vi "Autonomous Independent.vi"() -> ()   [LabVIEW 2013]
doc: "This VI is called when autonomous begins, and will automatically be terminated when autonomous ends. You can carry out timed or sensor driven robot movement independently without needing to return to the caller."
uses:
  Robot Global Data.vi
  <vilib>/Rock Robotics/WPI/RobotDrive/WPI_RobotDriveArcadeDrive_Standard(NoSaturation).vi
panel:
  out "Limit Switch":bool
  out "Light on if Arm is Down/Going Down":bool
  out "Intake pneumatics":bool
  out "Drive Right Motor":dbl
  out "Drive Left Motor":dbl
  # "Be sure to right-click and choose Data Operations>>Make Current Value default if you want to save the array values with the VI"
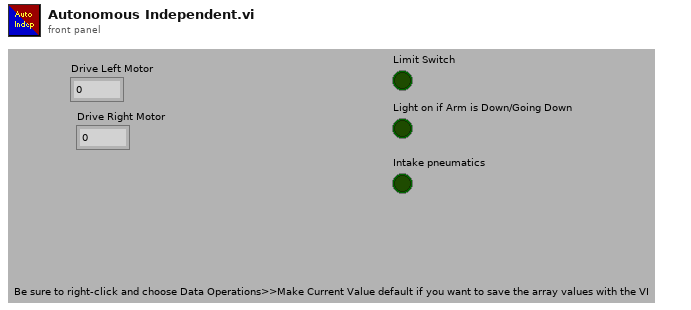
[diagram p1: front panel]
types:
  T1 = typedef "WPI_RobotDriveDevRef.ctl" = cluster{"DevStatus":errorcluster, "Motors[]":T2[], "Square Inputs":bool, "Max Output":dbl, "Isochronous":bool}
  T2 = typedef "WPI_MotorControlDeviceRef.ctl" = cluster{"DeviceStatus":errorcluster, "Type":enum16{"PWM", "CAN"}, "PWM":cluster{"Digital Module":T3, "PWM Channel":T4, "DeadBand":T5}, "CAN":cluster{"Device Number":u8, "Control Mode":T6, "Semaphore":T7, "Max Vout":dbl}, "Invert":bool, "TransformRef":T8, "InvTransformRef":T8}
  T3 = typedef "FPGA_TypedefDigitalModule.ctl" = enum16{"Digital Module 1", "Digital Module 2"}
  T4 = typedef "FPGA_DIOPWMChannel.ctl" = enum8{"PWM 1", "PWM 2", "PWM 3", "PWM 4", "PWM 5", "PWM 6", "PWM 7", "PWM 8", "PWM 9", "PWM 10", "Invalid"}
  T5 = typedef "WPI_PWMDeadband.ctl" = cluster{"Name":string, "maxPositivePwm":i32, "minPositivePwm":i32, "centerPwm":i32, "maxNegativePwm":i32, "minNegativePwm":i32, "angularRange":u16}
  T6 = typedef "WPI_CANJaguar_ControlMode.ctl" = enum8{"Percent VBus", "Current", "Speed", "Position", "Voltage"}
  T7 = typedef "Semaphore RefNum" = refnum<k1>
  T8 = typedef "WPI_PWMTransform_ConPane.ctl" = refnum<vi>
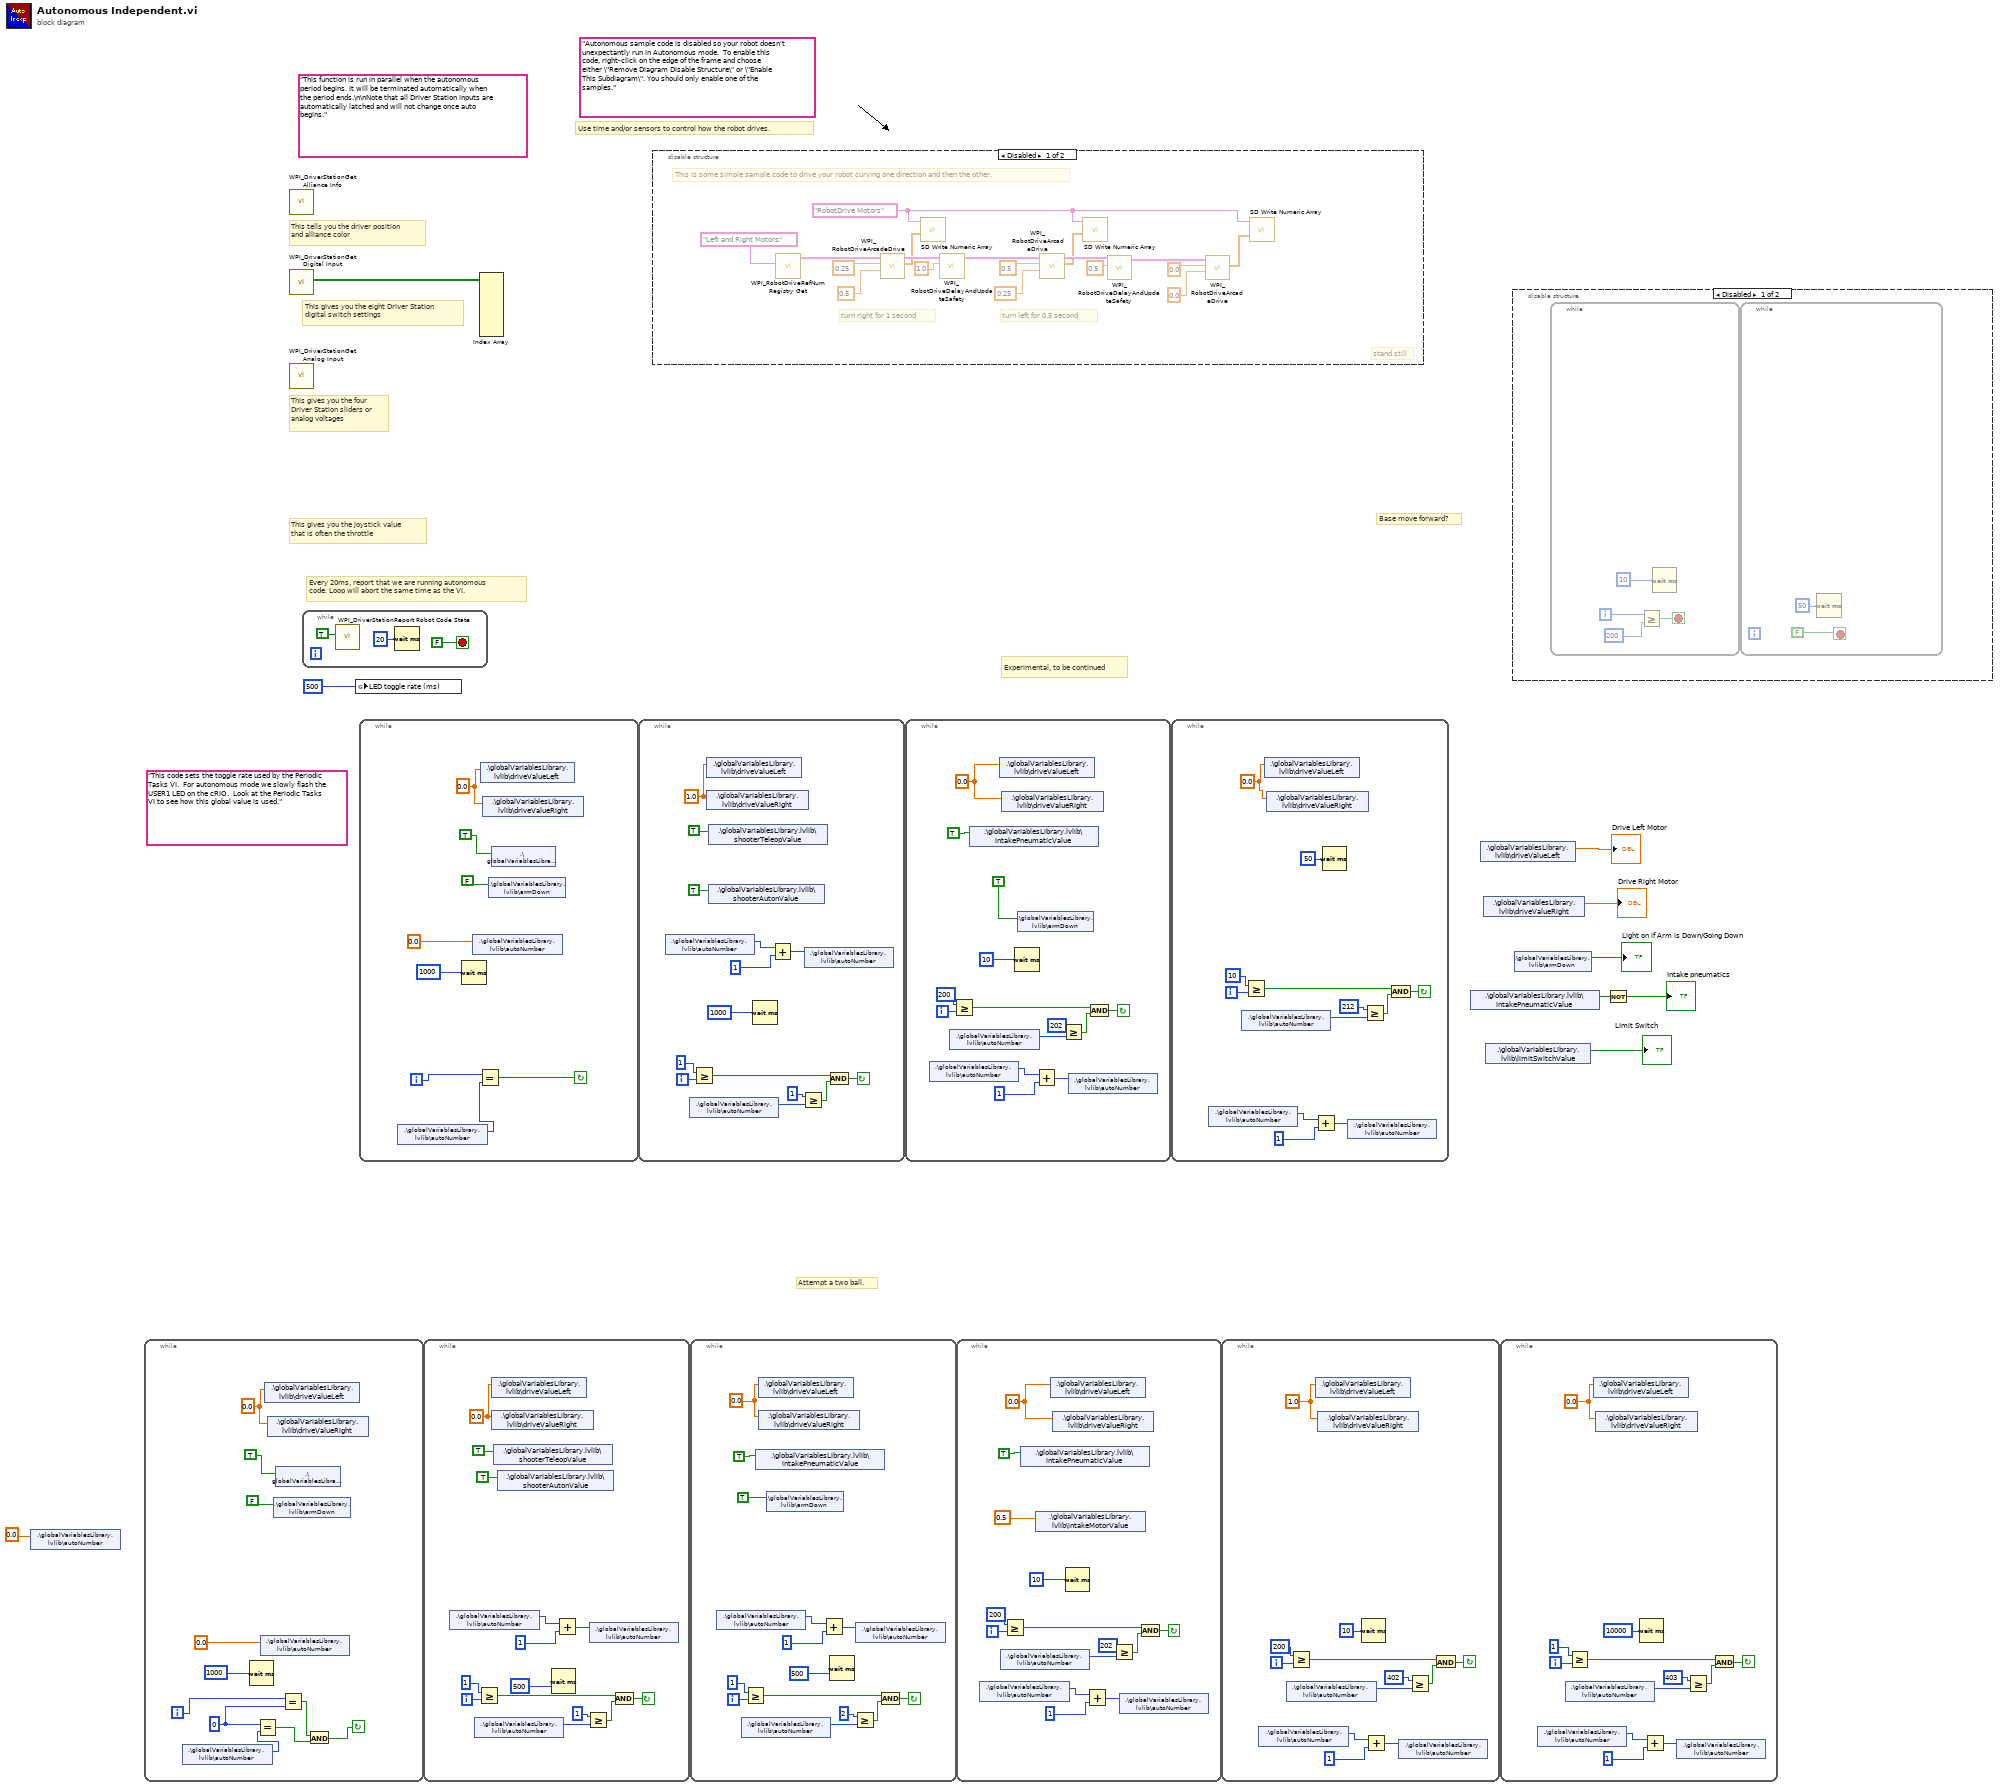
[diagram p0: block diagram]
diagram:
  (unwired) "This code sets the toggle rate used by the Periodic Tasks VI.  For autonomous mode we slowly flash the USER1 LED on the cRIO.  Look at the Periodic Tasks VI to see how this global value is used."
  (unwired) "Autonomous sample code is disabled so your robot doesn't unexpectantly run in Autonomous mode.  To enable this code, right-click on the edge of the frame and choose either \"Remove Diagram Disable Structure\" or \"Enable This Subdiagram\". You should only enable one of the samples."
  (unwired) "This function is run in parallel when the autonomous period begins. It will be terminated automatically when the period ends.\n\nNote that all Driver Station inputs are automatically latched and will not change once auto begins."
  # "Attempt a two ball."
  # "Base move forward?"
  # "Experimental, to be continued"
  # "Every 20ms, report that we are running autonomous\ncode. Loop will abort the same time as the VI."
  # "This gives you the joystick value\nthat is often the throttle"
  # "Use time and/or sensors to control how the robot drives."
  # "This tells you the driver position\nand alliance color"
  # "This gives you the eight Driver Station\ndigital switch settings"
  # "This gives you the four\nDriver Station sliders or\nanalog voltages"
  n1 = shared-variable ".\\globalVariablesLibrary.lvlib\\autoNumber"(0.0) -> ()  [unwired: 1 in, 1 out]
  n2 = while {
    i -> [w13]
    stop <- w14 continue-if-true
    w11 = 0
    w19 = 0.0
    n3 = shared-variable ".\\globalVariablesLibrary.lvlib\\autoNumber"() -> (w15:i16)  [unwired: 1 in, 1 out]
    n4 = Wait (ms)(milliseconds to wait=u32 1000) -> ()  [unwired: 1 out]
    n5 = Equal?(x=w11, y=w15) -> (x = y?=w10:bool)
    n6 = shared-variable ".\\globalVariablesLibrary.lvlib\\autoNumber"(0.0) -> ()  [unwired: 1 in, 1 out]
    n7 = shared-variable ".\\globalVariablesLibrary.lvlib\\driveValueLeft"(w19) -> ()  [unwired: 1 in, 1 out]
    n8 = shared-variable ".\\globalVariablesLibrary.lvlib\\driveValueRight"(w19) -> ()  [unwired: 1 in, 1 out]
    n9 = shared-variable ".\\globalVariablesLibrary.lvlib\\armDown"(FALSE) -> ()  [unwired: 1 in, 1 out]
    n10 = shared-variable ".\\globalVariablesLibrary.lvlib\\armUp"(TRUE) -> ()  [unwired: 1 in, 1 out]
    n11 = Equal?(x=w13, y=w11) -> (x = y?=w12:bool)
    n12 = And(x=w12, y=w10) -> (x .and. y?=w14:bool)
  }
  n13 = call <vilib>:"WPI_DriverStationGet Alliance Info.vi"() -> ()  [unwired: 12 out]
  n14 = call <vilib>:"WPI_DriverStationGet Digital Input.vi"() -> ("Driver Station Digital Input (1-8)"=w9:bool[])  [unwired: 11 out]
  n15 = call <vilib>:"WPI_DriverStationGet Analog Input.vi"() -> ()  [unwired: 12 out]
  n16 = while {
    stop <- FALSE stop-if-true
    n17 = call <vilib>:"WPI_DriverStationReport Robot Code State.vi"("Autonomous"=TRUE) -> ()  [unwired: 10 in, 1 out]
    n18 = Wait (ms)(milliseconds to wait=u32 20) -> ()  [unwired: 1 out]
  }
  n19 = global write "Robot Global Data.vi" "LED toggle rate (ms)"(u32 500 ("LED ms toggle rate")) -> ()
  n20 = while {
    i -> [w25]
    stop <- w24 continue-if-true
    w30 = 0.0
    n21 = shared-variable ".\\globalVariablesLibrary.lvlib\\autoNumber"() -> (w26:i16)  [unwired: 1 in, 1 out]
    n22 = Wait (ms)(milliseconds to wait=u32 1000) -> ()  [unwired: 1 out]
    n23 = shared-variable ".\\globalVariablesLibrary.lvlib\\autoNumber"(0.0) -> ()  [unwired: 1 in, 1 out]
    n24 = Equal?(x=w25, y=w26) -> (x = y?=w24:bool)
    n25 = shared-variable ".\\globalVariablesLibrary.lvlib\\driveValueLeft"(w30) -> ()  [unwired: 1 in, 1 out]
    n26 = shared-variable ".\\globalVariablesLibrary.lvlib\\driveValueRight"(w30) -> ()  [unwired: 1 in, 1 out]
    n27 = shared-variable ".\\globalVariablesLibrary.lvlib\\armDown"(FALSE) -> ()  [unwired: 1 in, 1 out]
    n28 = shared-variable ".\\globalVariablesLibrary.lvlib\\armUp"(TRUE) -> ()  [unwired: 1 in, 1 out]
  }
  n29 = while {
    i -> [w35]
    stop <- w32 continue-if-true
    w42 = 0.0
    n30 = shared-variable ".\\globalVariablesLibrary.lvlib\\autoNumber"() -> (w41:i16)  [unwired: 1 in, 1 out]
    n31 = shared-variable ".\\globalVariablesLibrary.lvlib\\autoNumber"() -> (w38:i16)  [unwired: 1 in, 1 out]
    n32 = Greater Or Equal?(x=1, y=w35) -> (x >= y?=w33:bool)
    n33 = shared-variable ".\\globalVariablesLibrary.lvlib\\driveValueLeft"(w42) -> ()  [unwired: 1 in, 1 out]
    n34 = shared-variable ".\\globalVariablesLibrary.lvlib\\driveValueRight"(w42) -> ()  [unwired: 1 in, 1 out]
    n35 = shared-variable ".\\globalVariablesLibrary.lvlib\\shooterTeleopValue"(TRUE) -> ()  [unwired: 1 in, 1 out]
    n36 = shared-variable ".\\globalVariablesLibrary.lvlib\\shooterAutonValue"(TRUE) -> ()  [unwired: 1 in, 1 out]
    n37 = Wait (ms)(milliseconds to wait=u32 500) -> ()  [unwired: 1 out]
    n38 = Add(x=w41, y=1) -> (x+y=w40:i32)
    n39 = Greater Or Equal?(x=1, y=w38) -> (x >= y?=w36:bool)
    n40 = shared-variable ".\\globalVariablesLibrary.lvlib\\autoNumber"(w40) -> ()  [unwired: 1 in, 1 out]
    n41 = And(x=w33, y=w36) -> (x .and. y?=w32:bool)
  }
  n42 = Index Array(array=w9) -> ()  [unwired: 8 in, 8 out]
  n43 = while {
    i -> [w49]
    stop <- w46 continue-if-true
    w56 = 1.0
    n44 = shared-variable ".\\globalVariablesLibrary.lvlib\\autoNumber"() -> (w55:i16)  [unwired: 1 in, 1 out]
    n45 = shared-variable ".\\globalVariablesLibrary.lvlib\\autoNumber"() -> (w52:i16)  [unwired: 1 in, 1 out]
    n46 = Greater Or Equal?(x=1, y=w49) -> (x >= y?=w47:bool)
    n47 = shared-variable ".\\globalVariablesLibrary.lvlib\\driveValueLeft"(w56) -> ()  [unwired: 1 in, 1 out]
    n48 = shared-variable ".\\globalVariablesLibrary.lvlib\\driveValueRight"(w56) -> ()  [unwired: 1 in, 1 out]
    n49 = shared-variable ".\\globalVariablesLibrary.lvlib\\shooterTeleopValue"(TRUE) -> ()  [unwired: 1 in, 1 out]
    n50 = shared-variable ".\\globalVariablesLibrary.lvlib\\shooterAutonValue"(TRUE) -> ()  [unwired: 1 in, 1 out]
    n51 = Wait (ms)(milliseconds to wait=u32 1000) -> ()  [unwired: 1 out]
    n52 = Add(x=w55, y=1) -> (x+y=w54:i32)
    n53 = Greater Or Equal?(x=1, y=w52) -> (x >= y?=w50:bool)
    n54 = shared-variable ".\\globalVariablesLibrary.lvlib\\autoNumber"(w54) -> ()  [unwired: 1 in, 1 out]
    n55 = And(x=w47, y=w50) -> (x .and. y?=w46:bool)
  }
  n56 = disable-structure shown="Disabled" {
    frame Disabled {
      w60 = "RobotDrive Motors" ("Name")
      # "This is some simple sample code to drive your robot curving one direction and then the other."
      # "stand still"
      # "turn left for 0.5 second"
      # "turn right for 1 second"
      n57 = call <vilib>:"WPI_RobotDriveRefNum Registry Get.vi"("refnum name"="Left and Right Motors") -> ("RobotDriveDevRef"=w64:T1)  [unwired: 1 in, 9 out]
      n58 = call-poly <vilib>:"WPI_RobotDriveArcadeDrive.vi"("Y axis value"=0.5 ("X axis value"), "X axis value"=0.25, "RobotDriveDevRef"=w64) -> ("Motor Values"=w63:dbl[], "RobotDriveDevRef"=w71:T1)  [unwired: 1 in, 6 out]
      n59 = call <vilib>:"SD Write Numeric Array.vi"("Numeric Array"=w63, "Name"=w60) -> ()  [unwired: 8 in, 2 out]
      n60 = call <vilib>:"WPI_RobotDriveDelayAndUpdateSafety.vi"("Delay (s)"=1.0, "RobotDriveDevRef"=w71) -> ("RobotDriveDevRef 2"=w70:T1)  [unwired: 8 in, 1 out]
      n61 = call-poly <vilib>:"WPI_RobotDriveArcadeDrive.vi"("Y axis value"=0.25 ("X axis value"), "X axis value"=0.5, "RobotDriveDevRef"=w70) -> ("Motor Values"=w62:dbl[], "RobotDriveDevRef"=w69:T1)  [unwired: 1 in, 6 out]
      n62 = call <vilib>:"SD Write Numeric Array.vi"("Numeric Array"=w62, "Name"=w60) -> ()  [unwired: 8 in, 2 out]
      n63 = call <vilib>:"WPI_RobotDriveDelayAndUpdateSafety.vi"("Delay (s)"=0.5, "RobotDriveDevRef"=w69) -> ("RobotDriveDevRef 2"=w68:T1)  [unwired: 8 in, 1 out]
      n64 = call-poly <vilib>:"WPI_RobotDriveArcadeDrive.vi"("Y axis value"=0.0 ("X axis value"), "X axis value"=0.0, "RobotDriveDevRef"=w68) -> ("Motor Values"=w61:dbl[])  [unwired: 1 in, 7 out]
      n65 = call <vilib>:"SD Write Numeric Array.vi"("Numeric Array"=w61, "Name"=w60) -> ()  [unwired: 8 in, 2 out]
    }
    frame Enabled {
    }
  }
  n66 = while {
    i -> [w83]
    stop <- w80 continue-if-true
    w90 = 0.0
    n67 = shared-variable ".\\globalVariablesLibrary.lvlib\\autoNumber"() -> (w89:i16)  [unwired: 1 in, 1 out]
    n68 = shared-variable ".\\globalVariablesLibrary.lvlib\\autoNumber"() -> (w86:i16)  [unwired: 1 in, 1 out]
    n69 = Greater Or Equal?(x=1, y=w83) -> (x >= y?=w81:bool)
    n70 = shared-variable ".\\globalVariablesLibrary.lvlib\\intakePneumaticValue"(TRUE) -> ()  [unwired: 1 in, 1 out]
    n71 = shared-variable ".\\globalVariablesLibrary.lvlib\\driveValueLeft"(w90) -> ()  [unwired: 1 in, 1 out]
    n72 = shared-variable ".\\globalVariablesLibrary.lvlib\\driveValueRight"(w90) -> ()  [unwired: 1 in, 1 out]
    n73 = shared-variable ".\\globalVariablesLibrary.lvlib\\armDown"(TRUE) -> ()  [unwired: 1 in, 1 out]
    n74 = Add(x=w89, y=1) -> (x+y=w88:i32)
    n75 = Wait (ms)(milliseconds to wait=u32 500) -> ()  [unwired: 1 out]
    n76 = Greater Or Equal?(x=2, y=w86) -> (x >= y?=w84:bool)
    n77 = shared-variable ".\\globalVariablesLibrary.lvlib\\autoNumber"(w88) -> ()  [unwired: 1 in, 1 out]
    n78 = And(x=w81, y=w84) -> (x .and. y?=w80:bool)
  }
  n79 = while {
    i -> [w96]
    stop <- w95 continue-if-true
    w103 = 0.0 ("Output")
    n80 = shared-variable ".\\globalVariablesLibrary.lvlib\\autoNumber"() -> (w94:i16)  [unwired: 1 in, 1 out]
    n81 = shared-variable ".\\globalVariablesLibrary.lvlib\\autoNumber"() -> (w101:i16)  [unwired: 1 in, 1 out]
    n82 = Greater Or Equal?(x=200, y=w96) -> (x >= y?=w97:bool)
    n83 = shared-variable ".\\globalVariablesLibrary.lvlib\\intakePneumaticValue"(TRUE) -> ()  [unwired: 1 in, 1 out]
    n84 = shared-variable ".\\globalVariablesLibrary.lvlib\\driveValueLeft"(w103) -> ()  [unwired: 1 in, 1 out]
    n85 = shared-variable ".\\globalVariablesLibrary.lvlib\\driveValueRight"(w103) -> ()  [unwired: 1 in, 1 out]
    n86 = Wait (ms)(milliseconds to wait=u32 10) -> ()  [unwired: 1 out]
    n87 = shared-variable ".\\globalVariablesLibrary.lvlib\\armDown"(TRUE) -> ()  [unwired: 1 in, 1 out]
    n88 = Add(x=w94, y=1) -> (x+y=w93:i32)
    n89 = Greater Or Equal?(x=202, y=w101) -> (x >= y?=w99:bool)
    n90 = shared-variable ".\\globalVariablesLibrary.lvlib\\autoNumber"(w93) -> ()  [unwired: 1 in, 1 out]
    n91 = And(x=w97, y=w99) -> (x .and. y?=w95:bool)
  }
  n92 = while {
    i -> [w111]
    stop <- w110 continue-if-true
    w117 = 0.0 ("Output")
    n93 = shared-variable ".\\globalVariablesLibrary.lvlib\\autoNumber"() -> (w109:i16)  [unwired: 1 in, 1 out]
    n94 = shared-variable ".\\globalVariablesLibrary.lvlib\\autoNumber"() -> (w116:i16)  [unwired: 1 in, 1 out]
    n95 = Greater Or Equal?(x=200, y=w111) -> (x >= y?=w112:bool)
    n96 = shared-variable ".\\globalVariablesLibrary.lvlib\\intakePneumaticValue"(TRUE) -> ()  [unwired: 1 in, 1 out]
    n97 = shared-variable ".\\globalVariablesLibrary.lvlib\\intakeMotorValue"(0.5) -> ()  [unwired: 1 in, 1 out]
    n98 = shared-variable ".\\globalVariablesLibrary.lvlib\\driveValueLeft"(w117) -> ()  [unwired: 1 in, 1 out]
    n99 = shared-variable ".\\globalVariablesLibrary.lvlib\\driveValueRight"(w117) -> ()  [unwired: 1 in, 1 out]
    n100 = Wait (ms)(milliseconds to wait=u32 10) -> ()  [unwired: 1 out]
    n101 = Add(x=w109, y=1) -> (x+y=w108:i32)
    n102 = Greater Or Equal?(x=202, y=w116) -> (x >= y?=w114:bool)
    n103 = shared-variable ".\\globalVariablesLibrary.lvlib\\autoNumber"(w108) -> ()  [unwired: 1 in, 1 out]
    n104 = And(x=w112, y=w114) -> (x .and. y?=w110:bool)
  }
  n105 = while {
    i -> [w123]
    stop <- w124 continue-if-true
    w130 = 0.0
    n106 = shared-variable ".\\globalVariablesLibrary.lvlib\\autoNumber"() -> (w122:i16)  [unwired: 1 in, 1 out]
    n107 = shared-variable ".\\globalVariablesLibrary.lvlib\\autoNumber"() -> (w129:i16)  [unwired: 1 in, 1 out]
    n108 = Greater Or Equal?(x=10, y=w123) -> (x >= y?=w125:bool)
    n109 = shared-variable ".\\globalVariablesLibrary.lvlib\\driveValueLeft"(w130) -> ()  [unwired: 1 in, 1 out]
    n110 = shared-variable ".\\globalVariablesLibrary.lvlib\\driveValueRight"(w130) -> ()  [unwired: 1 in, 1 out]
    n111 = Add(x=w122, y=1) -> (x+y=w121:i32)
    n112 = Wait (ms)(milliseconds to wait=u32 50) -> ()  [unwired: 1 out]
    n113 = shared-variable ".\\globalVariablesLibrary.lvlib\\autoNumber"(w121) -> ()  [unwired: 1 in, 1 out]
    n114 = Greater Or Equal?(x=212, y=w129) -> (x >= y?=w127:bool)
    n115 = And(x=w125, y=w127) -> (x .and. y?=w124:bool)
  }
  n116 = while {
    i -> [w135]
    stop <- w136 continue-if-true
    w142 = 1.0
    n117 = shared-variable ".\\globalVariablesLibrary.lvlib\\autoNumber"() -> (w134:i16)  [unwired: 1 in, 1 out]
    n118 = shared-variable ".\\globalVariablesLibrary.lvlib\\autoNumber"() -> (w141:i16)  [unwired: 1 in, 1 out]
    n119 = Greater Or Equal?(x=200, y=w135) -> (x >= y?=w137:bool)
    n120 = shared-variable ".\\globalVariablesLibrary.lvlib\\driveValueLeft"(w142) -> ()  [unwired: 1 in, 1 out]
    n121 = shared-variable ".\\globalVariablesLibrary.lvlib\\driveValueRight"(w142) -> ()  [unwired: 1 in, 1 out]
    n122 = Wait (ms)(milliseconds to wait=u32 10) -> ()  [unwired: 1 out]
    n123 = Add(x=w134, y=1) -> (x+y=w133:i32)
    n124 = shared-variable ".\\globalVariablesLibrary.lvlib\\autoNumber"(w133) -> ()  [unwired: 1 in, 1 out]
    n125 = Greater Or Equal?(x=402, y=w141) -> (x >= y?=w139:bool)
    n126 = And(x=w137, y=w139) -> (x .and. y?=w136:bool)
  }
  n127 = shared-variable ".\\globalVariablesLibrary.lvlib\\intakePneumaticValue"() -> (w4:bool)  [unwired: 1 in, 1 out]
  n128 = shared-variable ".\\globalVariablesLibrary.lvlib\\driveValueLeft"() -> (→"Drive Left Motor":dbl)  [unwired: 1 in, 1 out]
  n129 = shared-variable ".\\globalVariablesLibrary.lvlib\\driveValueRight"() -> (→"Drive Right Motor":dbl)  [unwired: 1 in, 1 out]
  n130 = shared-variable ".\\globalVariablesLibrary.lvlib\\limitSwitchValue"() -> (→"Limit Switch":bool)  [unwired: 1 in, 1 out]
  n131 = while {
    i -> [w147]
    stop <- w148 continue-if-true
    w154 = 0.0
    n132 = shared-variable ".\\globalVariablesLibrary.lvlib\\autoNumber"() -> (w146:i16)  [unwired: 1 in, 1 out]
    n133 = shared-variable ".\\globalVariablesLibrary.lvlib\\autoNumber"() -> (w153:i16)  [unwired: 1 in, 1 out]
    n134 = Greater Or Equal?(x=1, y=w147) -> (x >= y?=w149:bool)
    n135 = shared-variable ".\\globalVariablesLibrary.lvlib\\driveValueLeft"(w154) -> ()  [unwired: 1 in, 1 out]
    n136 = shared-variable ".\\globalVariablesLibrary.lvlib\\driveValueRight"(w154) -> ()  [unwired: 1 in, 1 out]
    n137 = Wait (ms)(milliseconds to wait=u32 10000) -> ()  [unwired: 1 out]
    n138 = Add(x=w146, y=1) -> (x+y=w145:i32)
    n139 = shared-variable ".\\globalVariablesLibrary.lvlib\\autoNumber"(w145) -> ()  [unwired: 1 in, 1 out]
    n140 = Greater Or Equal?(x=403, y=w153) -> (x >= y?=w151:bool)
    n141 = And(x=w149, y=w151) -> (x .and. y?=w148:bool)
  }
  n142 = disable-structure shown="Disabled" {
    frame Disabled {
      n143 = while {
        i -> [w160]
        stop <- w158 stop-if-true
        n144 = Greater Or Equal?(x=w160, y=200) -> (x >= y?=w158:bool)
        n145 = Wait (ms)(milliseconds to wait=u32 10) -> ()  [unwired: 1 out]
      }
      n146 = while {
        stop <- FALSE stop-if-true
        n147 = Wait (ms)(milliseconds to wait=u32 50) -> ()  [unwired: 1 out]
      }
    }
    frame Enabled {
    }
  }
  n148 = shared-variable ".\\globalVariablesLibrary.lvlib\\armDown"() -> (→"Light on if Arm is Down/Going Down":bool)  [unwired: 1 in, 1 out]
  n149 = Not(x=w4) -> (.not. x?=→"Intake pneumatics":bool)
